vi "Colorbox to RGB.vi"(1 "Color":u32) -> (0 "Material":T1)   [LabVIEW 2016]
uses:
  <vilib>/Utility/miscctls.llb/LVRGBAColorTypeDef.ctl
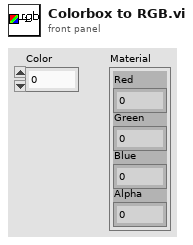
[diagram p1: front panel]
types:
  T1 = typedef "LVRGBAColorTypeDef.ctl" = cluster{"Red":sgl, "Green":sgl, "Blue":sgl, "Alpha":sgl}
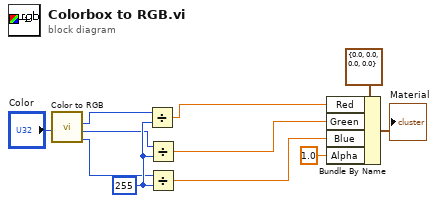
[diagram p0: block diagram]
diagram:
  w7 = u8 255 ("y")
  n1 = call <vilib>:"Color to RGB.vi"("Color"="Color") -> ("R"=w4:u8, "G"=w5:u8, "B"=w6:u8)  [unwired: 1 out]
  n2 = Divide(x=w4, y=w7) -> (x/y=w8:dbl)
  n3 = Divide(x=w5, y=w7) -> (x/y=w9:dbl)
  n4 = Divide(x=w6, y=w7) -> (x/y=w10:dbl)
  n5 = Bundle By Name(cluster=T1 {"Red"=0.0, "Green"=0.0, "Blue"=0.0, "Alpha"=0.0} ("Material:Diffuse"), "Red"=w8, "Green"=w9, "Blue"=w10, "Alpha"=sgl 1.0) -> (→"Material":T1)
